vi "M Solar cells.vi"(11 "EV3 in":T1) -> ()   [LabVIEW 2016]
uses:
  <vilib>/NXT/Subs/LVHSConnector.ctl
  <vilib>/NXT/LegoClasses/BrickReference/BrickReference.lvclass
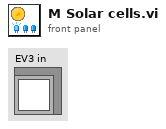
[diagram p1: front panel]
types:
  T1 = typedef "LVHSConnector.ctl" = refnum<class "BrickReference.lvclass">
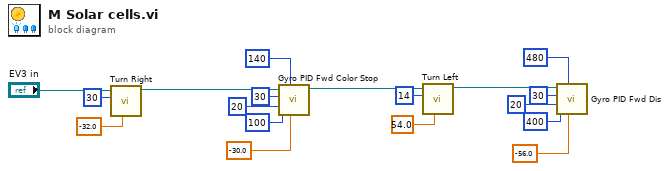
[diagram p0: block diagram]
diagram:
  n1 = call "Turn Right.vi"("Turning angle"=sgl -32.0, "Motor B (right)"=i8 30, "EV3 in"="EV3 in") -> ("EV3 out"=w15:T1)  [unwired: 8 in]
  n2 = call "Gyro PID Fwd Color Stop.vi"("Target angle"=sgl -30.0, "Threshold to Color"=140, "Threshold to slow"=100, "Min. speed"=20, "Max. speed"=30, "EV3 in"=w15) -> ("EV3 out"=w9:T1)  [unwired: 5 in]
  n3 = call "Turn Left.vi"("Turning angle"=sgl 54.0, "Motor B (right)"=i8 14, "EV3 in"=w9) -> ("EV3 out"=w6:T1)  [unwired: 8 in]
  n4 = call "Gyro PID Fwd Dis.vi"("Target angle"=sgl -56.0, "Threshold to stop"=480, "Threshold to slow"=400, "Min. speed"=20, "Max. speed"=30, "EV3 in"=w6) -> ()  [unwired: 5 in, 1 out]
